vi "EMV Flow Detector Minimum.vi"(8 "error in (no error)":errorcluster, 10 "ERD Data":T1, 11 ".NET Refnum in":refnum<k24>) -> (0 "error out":errorcluster, 2 "T7 Flow Dectection":bool, 3 ".NET Refnum out":refnum<k24>)   [LabVIEW 2016]
uses:
  Type Definitions/GEA3 HEWH ERD Data.ctl
  Type Definitions/GEA3 HEWH Mixing Valve.ctl
  C:/TechnologyLab/NI-2010/Drivers/GEA3 Toolkit/GEA3 DLL Source/GeaCommunication.dll
  GEA3 DLL Source/GeaCommunication.dll
panel:
  in  "Detection Slope":dbl=0.5 format="%#_13g"
  out "Slope Chart T7":dbl(graph)
  out "Current T7 Temperatures":dbl[](array[numeric])
  in  "T7_DELTA_FLOW_THRESHOLD":dbl=0.5
  # "reading now == 0\nreading in the past == 10"
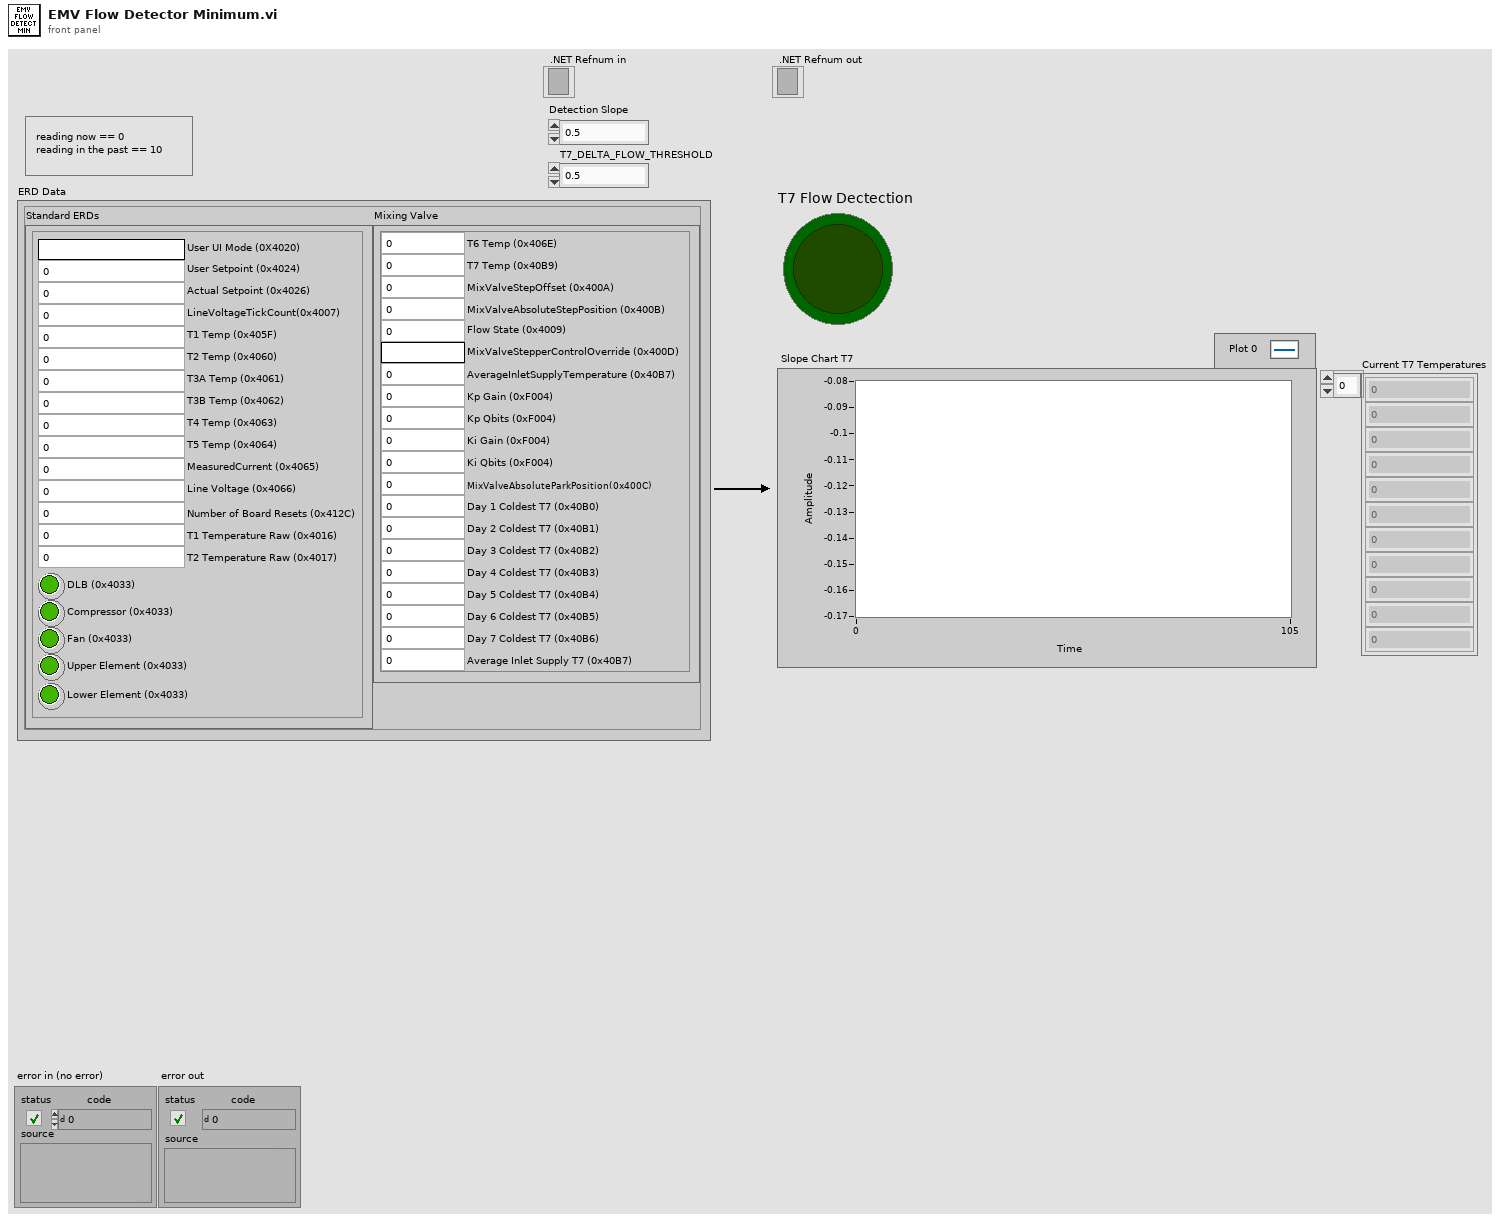
[diagram p1: front panel]
types:
  T1 = typedef "GEA3 HEWH ERD Data.ctl" = cluster{"Mixing Valve":T2, "Standard ERDs":cluster{"User UI Mode (0X4020)":string, "User Setpoint (0x4024)":u16, "Actual Setpoint (0x4026)":u16, "DLB (0x4033)":bool, "Compressor (0x4033)":bool, "Lower Element (0x4033)":bool, "Upper Element (0x4033)":bool, "Fan (0x4033)":bool, "T1 Temp (0x405F)":dbl, "T2 Temp (0x4060)":dbl, "T3A Temp (0x4061)":dbl, "T3B Temp (0x4062)":dbl, "T4 Temp (0x4063)":dbl, "T5 Temp (0x4064)":dbl, "Line Voltage (0x4066)":dbl, "MeasuredCurrent (0x4065)":dbl, "LineVoltageTickCount(0x4007)":u16, "Number of Board Resets (0x412C)":u16, "T1 Temperature Raw (0x4016)":u16, "T2 Temperature Raw (0x4017)":u16}}
  T2 = typedef "GEA3 HEWH Mixing Valve.ctl" = cluster{"T7 Temp (0x40B9)":dbl, "MixValveStepOffset (0x400A)":i16, "MixValveAbsoluteStepPosition (0x400B)":i16, "Flow State (0x4009)":u8, "MixValveStepperControlOverride (0x400D)":string, "AverageInletSupplyTemperature (0x40B7)":dbl, "T6 Temp (0x406E)":dbl, "Kp Gain (0xF004)":u16, "Kp Qbits (0xF004)":u16, "Ki Gain (0xF004)":u16, "Ki Qbits (0xF004)":u16, "MixValveAbsoluteParkPosition(0x400C)":i16, "Day 2 Coldest T7 (0x40B1)":dbl, "Day 1 Coldest T7 (0x40B0)":dbl, "Day 4 Coldest T7 (0x40B3)":dbl, "Day 3 Coldest T7 (0x40B2)":dbl, "Day 6 Coldest T7 (0x40B5)":dbl, "Day 5 Coldest T7 (0x40B4)":dbl, "Average Inlet Supply T7 (0x40B7)":dbl, "Day 7 Coldest T7 (0x40B6)":dbl}
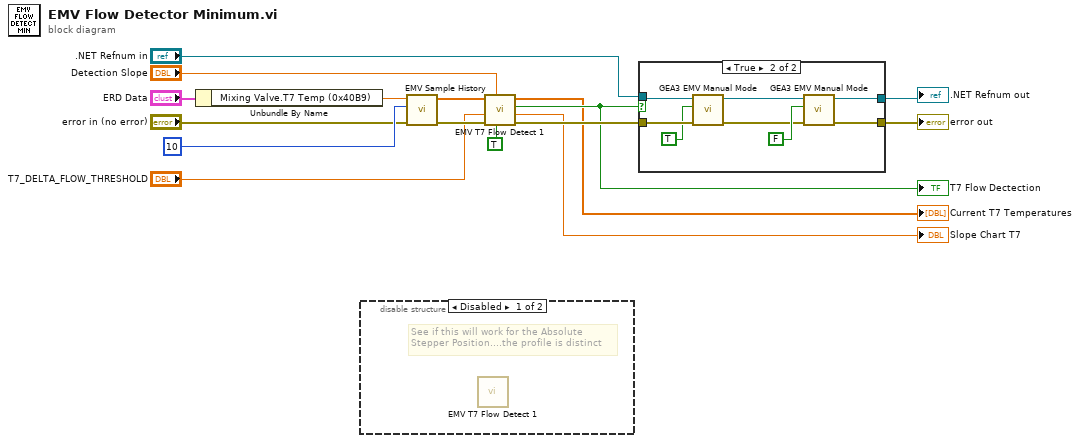
[diagram p0: block diagram]
diagram:
  n1 = Unbundle By Name("ERD Data") -> ("Mixing Valve.T7 Temp (0x40B9)"=w14:dbl)
  n2 = disable-structure shown="Disabled" {
    frame Disabled {
      # "See if this will work for the Absolute\nStepper Position....the profile is distinct"
      n3 = call "EMV T7 Flow Detect 1.vi"() -> ()  [unwired: 8 in, 4 out]
    }
    frame Enabled {
    }
  }
  n4 = call "EMV Sample History.vi"("error in (no error)"="error in (no error)", "length"=10, "T6 Temp"=w14) -> ("error out"=w12:errorcluster, "T6 History"=w13:dbl[])  [unwired: 7 in]
  n5 = call "EMV T7 Flow Detect 1.vi"("Detect Flow Start?"=TRUE, "Detection Slope"="Detection Slope", "error in (no error)"=w12, "T7_DELTA_FLOW_THRESHOLD"="T7_DELTA_FLOW_THRESHOLD", "Current T7 Temperatures"=w13) -> ("error out"=w4:errorcluster, "slope"=→"Slope Chart T7":dbl, "Detection?"=w3:bool, "Current T7 Temperatures Output"=→"Current T7 Temperatures":dbl[])  [unwired: 3 in]
  "T7 Flow Dectection" <- w3
  n6 = case shown="True" w3 {
    tunnel: w4 -> [w18 w26]
    tunnel: [w18 w24] -> w5
    tunnel: ".NET Refnum in" -> [w17 w25]
    tunnel: [w17 w23] -> w6
    frame False {
    }
    frame True {
      n7 = call "GEA3 EMV Manual Mode.vi"("error in (no error)"=w26, "Manual Mode?"=TRUE, ".NET Refnum in"=w25) -> ("error out"=w19:errorcluster, "GEA2 Reference Out"=w20:refnum<k24>)  [unwired: 7 in]
      n8 = call "GEA3 EMV Manual Mode.vi"("error in (no error)"=w19, "Manual Mode?"=FALSE, ".NET Refnum in"=w20) -> ("error out"=w24:errorcluster, "GEA2 Reference Out"=w23:refnum<k24>)  [unwired: 7 in]
    }
  }
  "error out" <- w5
  ".NET Refnum out" <- w6
